vi "dfd_Classical Order Estimation Specificaiton Conversion.vi"(7 "filter type":T2(ring), 8 "error in (no error)":errorcluster, 10 "ripple specs":T1={"passband"=0.1, "stopband"=40.0, "dB/linear? (T: dB)"=TRUE}, 11 "freq specs [Hz]":T3) -> (0 "error out":errorcluster, 1 "low cutoff freq: fl":dbl, 2 "high cutoff freq: fh":dbl, 3 "min transition band":dbl, 4 "A stop (dB)":dbl format="%.2f")   [LabVIEW 2017, in "NI_DigFilterLicensed.lvlib"]
uses:
  <vilib>/addons/Digital Filter Design/NI_DigFilterLicensed.lvlib
  <vilib>/addons/Digital Filter Design/_Objects.llb/DFD Filter Frequence Specification (Design).ctl
  <vilib>/addons/Digital Filter Design/_Objects.llb/DFD Filter Ripple Specification (Design).ctl
  <vilib>/addons/Digital Filter Design/NI_DigFilter_Design.lvlib
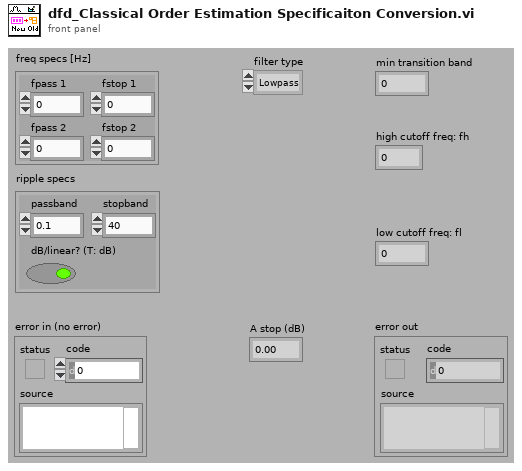
[diagram p1: front panel]
types:
  T1 = typedef "NI_DigFilterLicensed.lvlib/DFD Filter Ripple Specification (Design).ctl" = cluster{"passband":dbl, "stopband":dbl, "dB/linear? (T: dB)":bool}
  T2 = enum16{"Lowpass", "Highpass", "Bandpass", "Bandstop"}
  T3 = typedef "NI_DigFilterLicensed.lvlib/DFD Filter Frequence Specification (Design).ctl" = cluster{"fpass 1":dbl, "fstop 1":dbl, "fpass 2 ":dbl, "fstop 2":dbl}
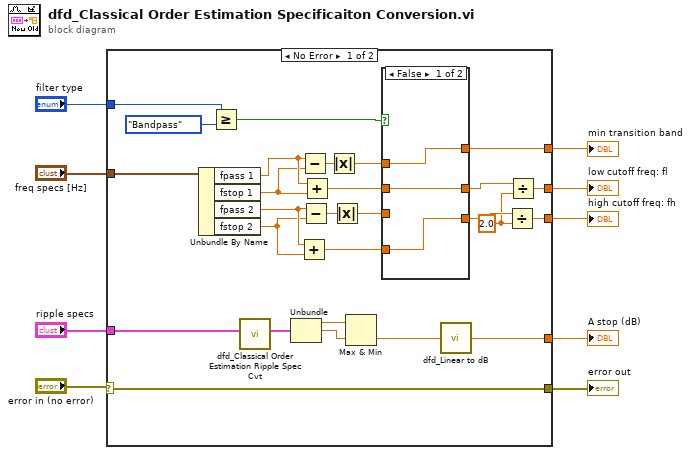
[diagram p0: block diagram]
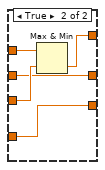
[diagram p2: hidden frame]
diagram:
  n1 = case shown="No Error" "error in (no error)" {
    selector: "error in (no error)" -> [w17 w45]
    tunnel: "freq specs [Hz]" -> [w36 _]
    tunnel: "filter type" -> [w34 _]
    tunnel: [w29 _] -> w7
    tunnel: "ripple specs" -> [w18 _]
    tunnel: [w10 _] -> w5
    tunnel: [w17 w45] -> w3
    tunnel: [w14 _] -> w2
    tunnel: [w13 _] -> w1
    frame No Error {
      w12 = 2.0 ("y")
      n2 = Unbundle By Name(w36) -> ("fpass 1"=w27:dbl, "fstop 1"=w26:dbl, "fpass 2"=w25:dbl, "fstop 2"=w24:dbl)
      n3 = Greater Or Equal?(x=w34, y=T2."Bandpass") -> (x >= y?=w32:bool)
      n4 = call <vilib>:"dfd_Classical Order Estimation Ripple Spec Cvt.vi"("ripple specs"=w18) -> ("ripple specs (linear)"=w19:T1)  [unwired: 10 out]
      n5 = Unbundle(w19) -> ("passband"=w21:dbl, "stopband"=w20:dbl)  [unwired: 1 out]
      n6 = Add(x=w25, y=w24) -> (x+y=w22:dbl)
      n7 = Subtract(x=w27, y=w26) -> (x-y=w35:dbl)
      n8 = Subtract(x=w25, y=w24) -> (x-y=w28:dbl)
      n9 = Add(x=w27, y=w26) -> (x+y=w23:dbl)
      n10 = Absolute Value(x=w35) -> (abs(x)=w31:dbl)
      n11 = Absolute Value(x=w28) -> (abs(x)=w30:dbl)
      n12 = Max & Min(x=w21, y=w20) -> (min(x,y)=w11:dbl)  [unwired: 1 out]
      n13 = case shown="False" w32 {
        tunnel: w31 -> [w39 w44]
        tunnel: w30 -> [_ w43]
        tunnel: [w39 w42] -> w29
        tunnel: w23 -> [w38 w40]
        tunnel: w22 -> [w37 w41]
        tunnel: [w37 w41] -> w15
        tunnel: [w38 w40] -> w16
        frame False {
        }
        frame True {
          n14 = Max & Min(x=w44, y=w43) -> (min(x,y)=w42:dbl)  [unwired: 1 out]
        }
      }
      n15 = call <vilib>:"dfd_Linear to dB.vi"("linear value"=w11) -> ("dB value"=w10:dbl)  [unwired: 1 in]
      n16 = Divide(x=w15, y=w12) -> (x/y=w13:dbl)
      n17 = Divide(x=w16, y=w12) -> (x/y=w14:dbl)
    }
    frame Error {
    }
  }
  "min transition band" <- w7
  "A stop (dB)" <- w5
  "error out" <- w3
  "low cutoff freq: fl" <- w2
  "high cutoff freq: fh" <- w1
